vi "Post_Method.vi"(6 "Headers":cluster{"Name":string, "Value":string}[](array[cluster]), 7 "Body Content-Type":string, 8 "error in (no error)":errorcluster, 9 "Body":string, 10 "Endpoint URL":string, 11 "Request in":refnum<class "Request.lvclass">) -> (0 "error out":errorcluster, 2 "Response out":refnum<class "Response.lvclass">, 3 "Request out":refnum<class "Request.lvclass">)   [LabVIEW 2020]
uses:
  Response/Response.lvclass
  Request/Request.lvclass
  Request/PowerShell_Format/Request_Control.ctl
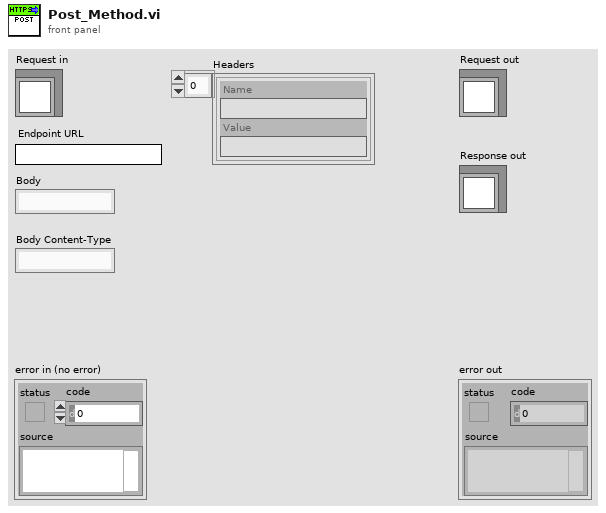
[diagram p1: front panel]
types:
  T1 = typedef "Request.lvclass/Request_Control.ctl" = enum16{"POST", "PATCH_MULTIPART", "POST_MULTIPART", "PATCH", "DELETE", "HEAD", "PUT", "GET"}
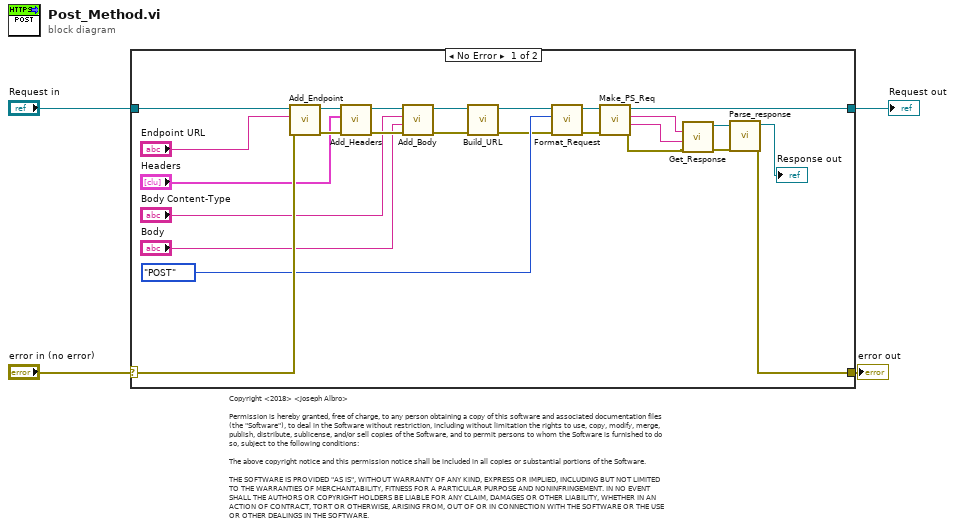
[diagram p0: block diagram]
diagram:
  # "Copyright <2018> <Joseph Albro>\n\nPermission is hereby granted, free of charge, to any person obtaining a copy of this software and associated documentation files (the \"Software\"), to deal in the Software without restriction, including without limitation the rights to use, copy, modify, merge, publish, distribute, sublicense, and/or sell copies of the Software, and to permit persons to whom the Software is furnished to do so, subject to the following conditions:\n\nThe above copyright notice and this permission notice shall be included in all copies or substantial portions of the Software.\n\nTHE SOFTWARE IS PROVIDED \"AS IS\", WITHOUT WARRANTY OF ANY KIND, EXPRESS OR IMPLIED, INCLUDING BUT NOT LIMITED TO THE WARRANTIES OF MERCHANTABILITY, FITNESS FOR A PARTICULAR PURPOSE AND NONINFRINGEMENT. IN NO EVENT SHALL THE AUTHORS OR COPYRIGHT HOLDERS BE LIABLE FOR ANY CLAIM, DAMAGES OR OTHER LIABILITY, WHETHER IN AN ACTION OF CONTRACT, TORT OR OTHERWISE, ARISING FROM, OUT OF OR IN CONNECTION WITH THE SOFTWARE OR THE USE OR OTHER DEALINGS IN THE SOFTWARE."
  n1 = case shown="No Error" "error in (no error)" {
    selector: "error in (no error)" -> [w25 w31]
    tunnel: [w15 w31] -> w3
    tunnel: [w27 w30] -> w1
    tunnel: "Request in" -> [w29 w30]
    frame No Error {
      n2 = call "Add_Endpoint.vi"("error in (no error)"=w25, "Endpoint URL"="Endpoint URL", "Request in"=w29) -> ("error out"=w26:errorcluster, "Request out"=w28:refnum<class "Request.lvclass">)  [unwired: 7 in]
      n3 = call "Add_Headers.vi"("error in (no error)"=w26, "Headers"="Headers", "Request in"=w28) -> ("error out"=w21:errorcluster, "Request out"=w22:refnum<class "Request.lvclass">)  [unwired: 7 in]
      n4 = call "Add_Body.vi"("error in (no error)"=w21, "Body"="Body", "Body Content-Type"="Body Content-Type", "Request in"=w22) -> ("error out"=w6:errorcluster, "Request out"=w8:refnum<class "Request.lvclass">)  [unwired: 6 in]
      n5 = call "Build_URL.vi"("error in (no error)"=w6, "Request in"=w8) -> ("error out"=w5:errorcluster, "Request out"=w7:refnum<class "Request.lvclass">)  [unwired: 8 in]
      n6 = call "Format_Request.vi"("error in (no error)"=w5, "Request"=Request_Control."POST", "Request in"=w7) -> ("error out"=w24:errorcluster, "Request out"=w23:refnum<class "Request.lvclass">)  [unwired: 7 in]
      n7 = call "Make_PS_Req.vi"("error in (no error)"=w24, "Request in"=w23) -> ("error out"=w16:errorcluster, "standard error"=w9:string, "standard output"=w17:string, "Request out"=w27:refnum<class "Request.lvclass">)  [unwired: 6 in]
      n8 = call "Get_Response.vi"("error in (no error)"=w16, "PS Error"=w9, "PS Response"=w17) -> ("error out"=w19:errorcluster, "Response out"=w20:refnum<class "Response.lvclass">)  [unwired: 7 in]
      n9 = call "Parse_response.vi"("error in (no error)"=w19, "Response in"=w20) -> ("error out"=w15:errorcluster, "Response out"=→"Response out":refnum<class "Response.lvclass">)  [unwired: 8 in]
    }
    frame Error {
    }
  }
  "error out" <- w3
  "Request out" <- w1
